vi "command to matlab.vi"(1 "matlabCommand":string) -> (0 "standard output":string)   [LabVIEW 2013]
panel:
  out "error out":errorcluster
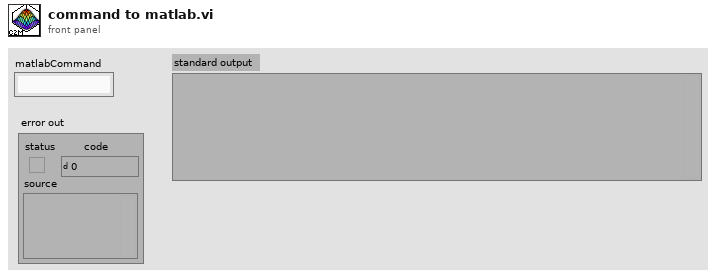
[diagram p1: front panel]
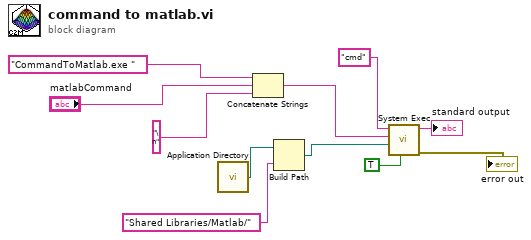
[diagram p0: block diagram]
diagram:
  n1 = call <vilib>:"Application Directory.vi"() -> ("Application Directory"=w3:path)
  n2 = Concatenate Strings("CommandToMatlab.exe " ("string"), "matlabCommand", "\n" ("string")) -> (w8:string)
  n3 = Build Path(base path=w3, name or relative path="Shared Libraries/Matlab/") -> (appended path=w1:path)
  n4 = call <vilib>:"System Exec.vi"("run minimized? (F)"=TRUE, "working directory"=w1, "standard input"=w8, "command line"="cmd") -> ("error out"=→"error out":errorcluster, "standard output"=→"standard output":string)  [unwired: 4 in, 2 out]
